vi "ntcp command.vi"(2 "error in":errorcluster, 3 "Input string":string="y\tdisplacement\t3.14\tz\trotation\t2.71828") -> (0 "Error out":errorcluster, 1 "NTCP Command":T1)   [LabVIEW 2009]
uses:
  Propose Command.ctl
panel:
  in  "Type":string[](array[string])=["displacement", "rotation", "force", "moment"]
  in  "Geometry":string[](array[string])=["x", "y", "z"]
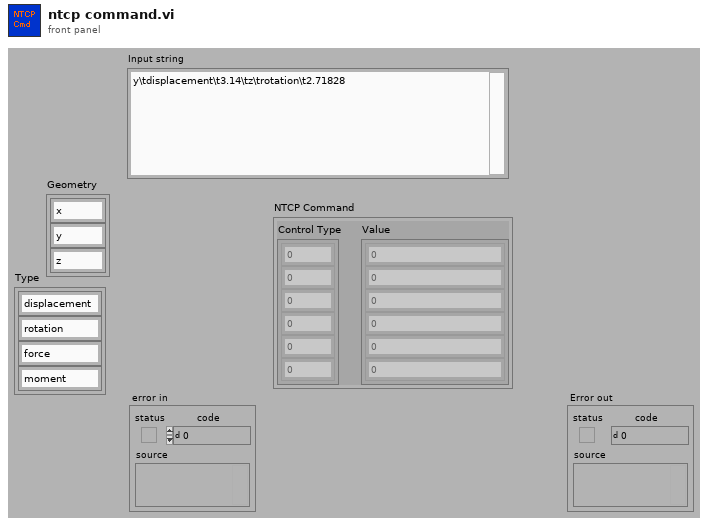
[diagram p1: front panel]
types:
  T1 = typedef "Propose Command.ctl" = cluster{"Control Type":i32[], "Value":dbl[]}
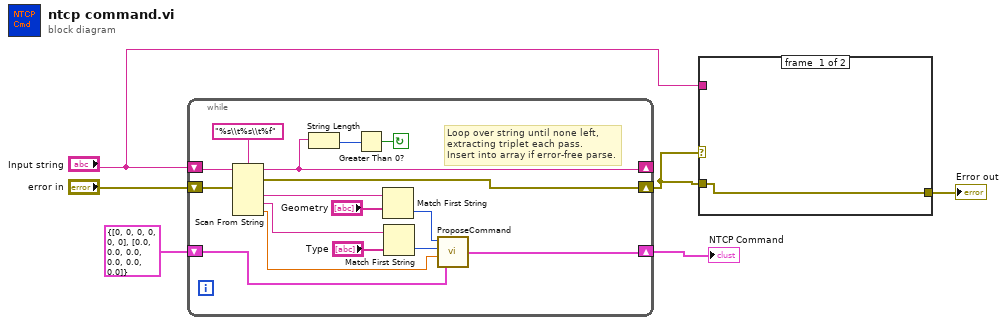
[diagram p0: block diagram]
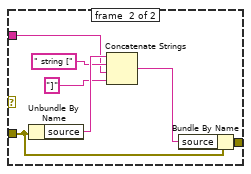
[diagram p2: hidden frame]
diagram:
  n1 = while {
    shift-right: [w18] -> _
    shift-left: "Input string" -> [w19]
    shift-right: [w8] -> w3
    shift-left: "error in" -> [w17]
    shift-right: [w9] -> w4
    shift-left: cluster{"Control Type":i32[], "Value":dbl[]} {"Control Type"=[0, 0, 0, 0, 0, 0], "Value"=[0.0, 0.0, 0.0, 0.0, 0.0, 0.0]} ("Incoming Command Cluster") -> [w7]
    stop <- w20 continue-if-true
    # "Loop over string until none left, \nextracting triplet each pass.\nInsert into array if error-free parse."
    n2 = Scan From String(format string="%s\\t%s\\t%f", input string=w19, error in=w17) -> (remaining string=w18:string, error out=w8:errorcluster, output 1=w16:string, output 2=w13:string, output 3=w10:dbl)  [unwired: 1 in, 4 out]
    n3 = String Length(string=w18) -> (length=w21:i32)
    n4 = Greater Than 0?(x=w21) -> (x > 0?=w20:bool)
    n5 = Match First String(2:"Geometry", 3:w16) -> (0:w12:i32)  [unwired: 1 out]
    n6 = Match First String(2:"Type", 3:w13) -> (0:w11:i32)  [unwired: 1 out]
    n7 = call "ProposeCommand.vi"("Incoming Command Cluster"=w7, "Value"=w10, "Type"=w11, "Geometry"=w12) -> ("Updated Command Cluster"=w9:T1)
  }
  "NTCP Command" <- w4
  n8 = case shown="Error" w3 {
    tunnel: w3 -> [w23 w25]
    tunnel: [w23 w26] -> w2
    tunnel: "Input string" -> [_ w28]
    frame #0 {
    }
    frame #1 {
      n9 = Unbundle By Name(w25) -> ("source"=w30:string)
      n10 = Concatenate Strings(w30, " string [" ("string"), w28, "]" ("string")) -> (w24:string)
      n11 = Bundle By Name(cluster=w25, "source"=w24) -> (w26:errorcluster)
    }
  }
  "Error out" <- w2
